vi "Begin.vi"() -> (0 "error out":errorcluster)   [LabVIEW 2013]
doc: "Called before other user functions, this VI is expected to open initial I/O refnums, load in file data, and do all program initialization. Notice that the <B>error out</B> terminal is simply used for data flow. Wiring it to other structures or subVIs ensures that this VI runs first."
uses:
  <vilib>/Rock Robotics/WPI/DriverStation/WPI_DriverStationRobotMode2.ctl
  <vilib>/Rock Robotics/WPI/Joystick/WPI_JoystickDeviceEnum.ctl
  <vilib>/Rock Robotics/SystemInterfaces/DIO/FPGA_DIOPWMChannel.ctl
  <vilib>/Rock Robotics/SystemInterfaces/AI/FPGA_AIGyroChannel.ctl
  <vilib>/Rock Robotics/SystemInterfaces/Typedef/FPGA_TypedefAnalogModuleForGyro.ctl
  <vilib>/Rock Robotics/SystemInterfaces/DIO/FPGA_DIOChannel.ctl
  <vilib>/Rock Robotics/SystemInterfaces/AI/FPGA_AIChannel.ctl
  <vilib>/Rock Robotics/SystemInterfaces/Typedef/FPGA_TypedefAnalogModule.ctl
  <vilib>/Rock Robotics/SystemInterfaces/Typedef/FPGA_TypedefDigitalModule.ctl
  Robot Global Data.vi
  <vilib>/Rock Robotics/WPI/MotorControl/WPI_MotorControlOpen Jaguar.vi
  <vilib>/Rock Robotics/WPI/MotorControl/WPI_MotorControlOpen Victor.vi
  <vilib>/Utility/file.llb/Read From Spreadsheet File (DBL).vi
panel:
  in  "file (use dialog)":path
  out "error out 3":errorcluster
  out "error out 2":errorcluster
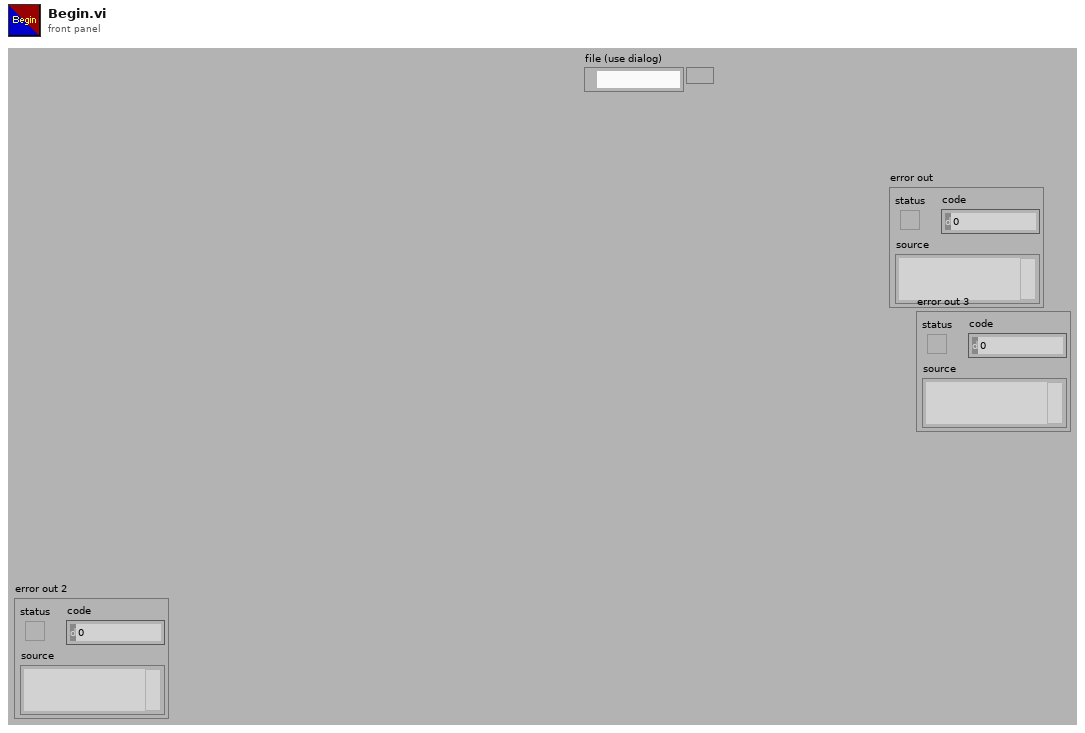
[diagram p1: front panel]
types:
  T1 = typedef "FPGA_TypedefAnalogModule.ctl" = enum16{"Analog Module 1", "Analog Module 2"}
  T2 = typedef "FPGA_AIChannel.ctl" = enum8{"AI 1", "AI 2", "AI 3", "AI 4", "AI 5", "AI 6", "AI 7", "AI 8", "Invalid"}
  T3 = typedef "FPGA_DIOChannel.ctl" = enum8{"DIO 1", "DIO 2", "DIO 3", "DIO 4", "DIO 5", "DIO 6", "DIO 7", "DIO 8", "DIO 9", "DIO 10", "DIO 11", "DIO 12", "DIO 13", "DIO 14", "Invalid"}
  T4 = typedef "FPGA_TypedefDigitalModule.ctl" = enum16{"Digital Module 1", "Digital Module 2"}
  T5 = typedef "FPGA_DIOPWMChannel.ctl" = enum8{"PWM 1", "PWM 2", "PWM 3", "PWM 4", "PWM 5", "PWM 6", "PWM 7", "PWM 8", "PWM 9", "PWM 10", "Invalid"}
  T6 = typedef "WPI_JoystickDeviceEnum.ctl" = enum16{"USB 1", "USB 2", "USB 3", "USB 4", "Kinect 1", "Kinect 2"}
  T7 = typedef "FPGA_TypedefAnalogModuleForGyro.ctl" = enum16{"Analog Module 1"}
  T8 = typedef "FPGA_AIGyroChannel.ctl" = enum8{"AI 1", "AI 2", "Invalid"}
  T9 = typedef "WPI_DriverStationRobotMode2.ctl" = enum16{"Autonomous Disabled", "Autonomous Enabled", "Teleop Disabled", "Teleop Enabled", "Timeout", "Finish", "Test Disabled", "Test Enabled"}
  T10 = typedef "WPI_JoystickDevRef.ctl" = cluster{"Device":T6}
  T11 = typedef "WPI_MotorControlDeviceRef.ctl" = cluster{"DeviceStatus":errorcluster, "Type":enum16{"PWM", "CAN"}, "PWM":cluster{"Digital Module":T4, "PWM Channel":T5, "DeadBand":T12}, "CAN":cluster{"Device Number":u8, "Control Mode":T13, "Semaphore":T14, "Max Vout":dbl}, "Invert":bool, "TransformRef":T15, "InvTransformRef":T15}
  T12 = typedef "WPI_PWMDeadband.ctl" = cluster{"Name":string, "maxPositivePwm":i32, "minPositivePwm":i32, "centerPwm":i32, "maxNegativePwm":i32, "minNegativePwm":i32, "angularRange":u16}
  T13 = typedef "WPI_CANJaguar_ControlMode.ctl" = enum8{"Percent VBus", "Current", "Speed", "Position", "Voltage"}
  T14 = typedef "Semaphore RefNum" = refnum<k1>
  T15 = typedef "WPI_PWMTransform_ConPane.ctl" = refnum<vi>
  T16 = typedef "WPI_ServoDeviceRef.ctl" = cluster{"DeviceStatus":errorcluster, "Digital Module":T4, "PWM Channel":T5, "DeadBand":T12}
  T17 = typedef "WPI_DigitalInputDevRef.ctl" = cluster{"DevStatus":errorcluster, "DIO Channel":T3, "Digital Module":T4}
  T18 = typedef "WPI_AnalogChannelDevRef.ctl" = cluster{"DevStatus":errorcluster, "Analog Module":T1, "Analog Channel":T2}
  T19 = typedef "WPI_GyroDevRef.ctl" = cluster{"DevStatus":errorcluster, "Analog Module":T1, "Analog Channel":T2, "Offset":dbl, "Gain (VoltsPerDegree/Second)":dbl}
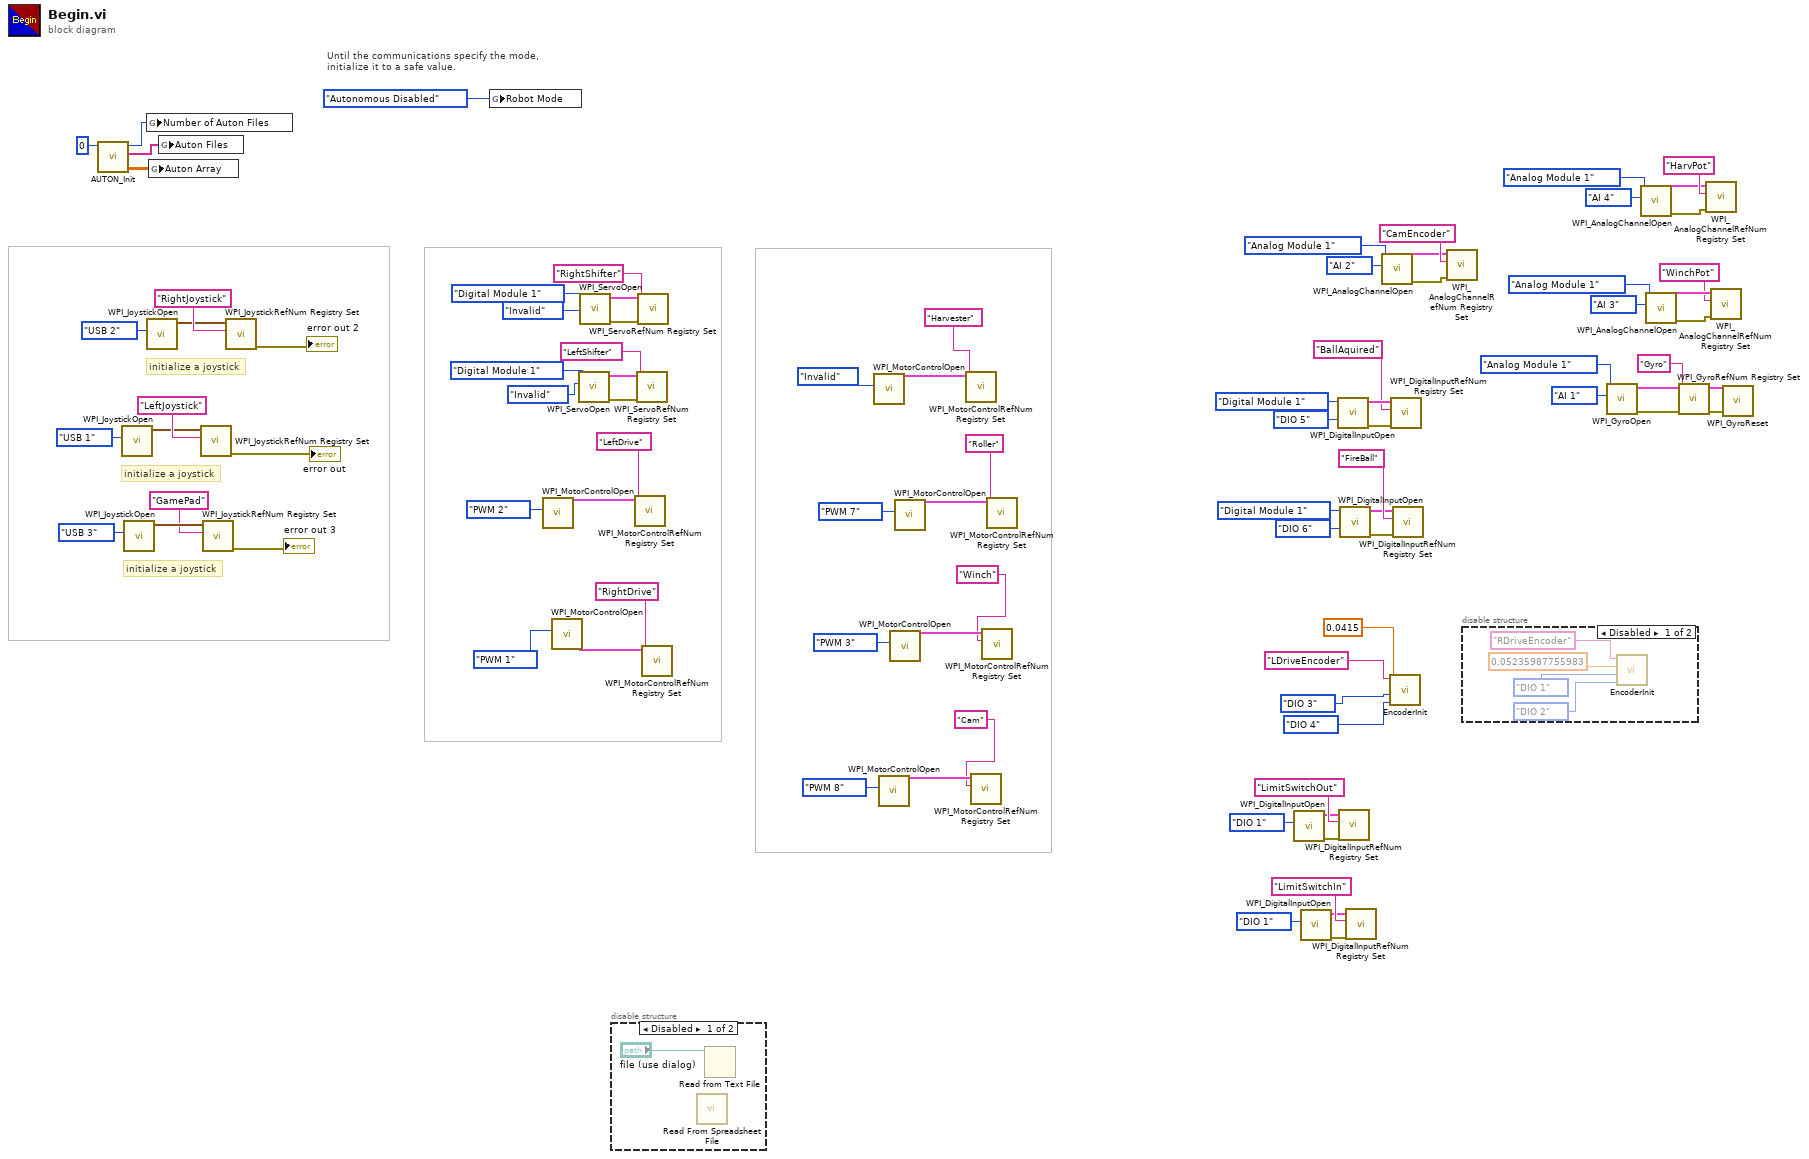
[diagram p0: block diagram]
diagram:
  # "initialize a joystick"
  # "initialize a joystick"
  # "initialize a joystick"
  # "Until the communications specify the mode,\ninitialize it to a safe value."
  n1 = call "AUTON_Init.vi"("Default File"=0) -> ("Auton Array"=w73:dbl[][], "Auton Files"=w72:string[], "Number of Auton Files"=w71:i64)  [unwired: 8 in]
  n2 = call <vilib>:"WPI_JoystickOpen.vi"("JoystickDevice"=WPI_JoystickDeviceEnum."USB 1") -> ("JoystickDevRef"=w87:T10)  [unwired: 10 in]
  n3 = call <vilib>:"WPI_JoystickOpen.vi"("JoystickDevice"=WPI_JoystickDeviceEnum."USB 3") -> ("JoystickDevRef"=w50:T10)  [unwired: 10 in]
  n4 = global write "Robot Global Data.vi" "Number of Auton Files"(w71) -> ()
  n5 = call <vilib>:"WPI_JoystickOpen.vi"("JoystickDevice"=WPI_JoystickDeviceEnum."USB 2") -> ("JoystickDevRef"=w83:T10)  [unwired: 10 in]
  n6 = global write "Robot Global Data.vi" "Auton Array"(w73) -> ()
  n7 = global write "Robot Global Data.vi" "Auton Files"(w72) -> ()
  n8 = call <vilib>:"WPI_JoystickRefNum Registry Set.vi"("refnum name"="LeftJoystick", "JoystickDevRef"=w87) -> ("error out"=→"error out":errorcluster)  [unwired: 8 in, 1 out]
  n9 = call <vilib>:"WPI_JoystickRefNum Registry Set.vi"("refnum name"="GamePad", "JoystickDevRef"=w50) -> ("error out"=→"error out 3":errorcluster)  [unwired: 8 in, 1 out]
  n10 = call <vilib>:"WPI_JoystickRefNum Registry Set.vi"("refnum name"="RightJoystick", "JoystickDevRef"=w83) -> ("error out"=→"error out 2":errorcluster)  [unwired: 8 in, 1 out]
  n11 = global write "Robot Global Data.vi" "Robot Mode"(WPI_DriverStationRobotMode2."Autonomous Disabled" ("Robot Mode")) -> ()
  n12 = call-poly <vilib>:"WPI_MotorControlOpen.vi"("PWM Channel"=FPGA_DIOPWMChannel."PWM 2") -> ("MotorControlDeviceRef"=w79:T11)  [unwired: 9 in, 1 out]
  n13 = call-poly <vilib>:"WPI_MotorControlOpen.vi"("PWM Channel"=FPGA_DIOPWMChannel."PWM 1") -> ("MotorControlDeviceRef"=w76:T11)  [unwired: 9 in, 1 out]
  n14 = call <vilib>:"WPI_ServoOpen.vi"("PWM Channel"=FPGA_DIOPWMChannel."Invalid", "Digital Module (Module 1)"=FPGA_TypedefDigitalModule."Digital Module 1") -> ("error out"=w40:errorcluster, "ServoDeviceRef"=w33:T16)  [unwired: 8 in]
  n15 = call <vilib>:"WPI_ServoOpen.vi"("PWM Channel"=FPGA_DIOPWMChannel."Invalid", "Digital Module (Module 1)"=FPGA_TypedefDigitalModule."Digital Module 1") -> ("error out"=w39:errorcluster, "ServoDeviceRef"=w38:T16)  [unwired: 8 in]
  n16 = disable-structure shown="Disabled" {
    frame Disabled {
      n17 = call-poly <vilib>:"Read From Spreadsheet File.vi"() -> ()  [unwired: 7 in, 5 out]
      n18 = Read from Text File(file (use dialog)="file (use dialog)") -> ()  [unwired: 3 in, 4 out]
    }
    frame Enabled {
    }
  }
  n19 = call <vilib>:"WPI_MotorControlRefNum Registry Set.vi"("refnum name"="LeftDrive", "MotorControlDevRef"=w79) -> ()  [unwired: 8 in, 2 out]
  n20 = call <vilib>:"WPI_ServoRefNum Registry Set.vi"("error in (no error)"=w40, "refnum name"="LeftShifter", "ServoDeviceRef"=w33) -> ()  [unwired: 7 in, 2 out]
  n21 = call <vilib>:"WPI_ServoRefNum Registry Set.vi"("error in (no error)"=w39, "refnum name"="RightShifter", "ServoDeviceRef"=w38) -> ()  [unwired: 7 in, 2 out]
  n22 = call <vilib>:"WPI_MotorControlRefNum Registry Set.vi"("refnum name"="RightDrive", "MotorControlDevRef"=w76) -> ()  [unwired: 8 in, 2 out]
  n23 = call-poly <vilib>:"WPI_MotorControlOpen.vi"("PWM Channel"=FPGA_DIOPWMChannel."Invalid") -> ("MotorControlDeviceRef"=w69:T11)  [unwired: 9 in, 1 out]
  n24 = call-poly <vilib>:"WPI_MotorControlOpen.vi"("PWM Channel"=FPGA_DIOPWMChannel."PWM 8") -> ("MotorControlDeviceRef"=w18:T11)  [unwired: 9 in, 1 out]
  n25 = call-poly <vilib>:"WPI_MotorControlOpen.vi"("PWM Channel"=FPGA_DIOPWMChannel."PWM 3") -> ("MotorControlDeviceRef"=w20:T11)  [unwired: 9 in, 1 out]
  n26 = call-poly <vilib>:"WPI_MotorControlOpen.vi"("PWM Channel"=FPGA_DIOPWMChannel."PWM 7") -> ("MotorControlDeviceRef"=w66:T11)  [unwired: 9 in, 1 out]
  n27 = call <vilib>:"WPI_MotorControlRefNum Registry Set.vi"("refnum name"="Harvester", "MotorControlDevRef"=w69) -> ()  [unwired: 8 in, 2 out]
  n28 = call <vilib>:"WPI_MotorControlRefNum Registry Set.vi"("refnum name"="Cam", "MotorControlDevRef"=w18) -> ()  [unwired: 8 in, 2 out]
  n29 = call <vilib>:"WPI_MotorControlRefNum Registry Set.vi"("refnum name"="Winch", "MotorControlDevRef"=w20) -> ()  [unwired: 8 in, 2 out]
  n30 = call <vilib>:"WPI_MotorControlRefNum Registry Set.vi"("refnum name"="Roller", "MotorControlDevRef"=w66) -> ()  [unwired: 8 in, 2 out]
  n31 = call <vilib>:"WPI_DigitalInputOpen.vi"("DIO Channel"=FPGA_DIOChannel."DIO 1") -> ("error out"=w22:errorcluster, "DigitalInputDevRef"=w23:T17)  [unwired: 9 in]
  n32 = call <vilib>:"WPI_DigitalInputOpen.vi"("DIO Channel"=FPGA_DIOChannel."DIO 1") -> ("error out"=w25:errorcluster, "DigitalInputDevRef"=w26:T17)  [unwired: 9 in]
  n33 = call <vilib>:"WPI_DigitalInputOpen.vi"("DIO Channel"=FPGA_DIOChannel."DIO 5", "Digital Module (Module 1)"=FPGA_TypedefDigitalModule."Digital Module 1") -> ("error out"=w60:errorcluster, "DigitalInputDevRef"=w59:T17)  [unwired: 8 in]
  n34 = call <vilib>:"WPI_DigitalInputRefNum Registry Set.vi"("error in (no error)"=w22, "refnum name"="LimitSwitchOut", "DigitalInputDevRef"=w23) -> ()  [unwired: 7 in, 2 out]
  n35 = call <vilib>:"WPI_DigitalInputOpen.vi"("DIO Channel"=FPGA_DIOChannel."DIO 6", "Digital Module (Module 1)"=FPGA_TypedefDigitalModule."Digital Module 1") -> ("error out"=w6:errorcluster, "DigitalInputDevRef"=w7:T17)  [unwired: 8 in]
  n36 = call <vilib>:"WPI_DigitalInputRefNum Registry Set.vi"("error in (no error)"=w25, "refnum name"="LimitSwitchIn", "DigitalInputDevRef"=w26) -> ()  [unwired: 7 in, 2 out]
  n37 = call <vilib>:"WPI_AnalogChannelOpen.vi"("Analog Channel"=FPGA_AIChannel."AI 2", "Analog Module (Module 1)"=FPGA_TypedefAnalogModule."Analog Module 1") -> ("error out"=w12:errorcluster, "AIDeviceRef"=w11:T18)  [unwired: 8 in]
  n38 = call "EncoderInit.vi"("refnum name"="LDriveEncoder", "DistancePerCount"=0.0415, "DIO Channel"=FPGA_DIOChannel."DIO 3", "DIO Channel 2"=FPGA_DIOChannel."DIO 4") -> ()  [unwired: 7 in]
  n39 = call <vilib>:"WPI_DigitalInputRefNum Registry Set.vi"("error in (no error)"=w60, "refnum name"="BallAquired", "DigitalInputDevRef"=w59) -> ()  [unwired: 7 in, 2 out]
  n40 = call <vilib>:"WPI_DigitalInputRefNum Registry Set.vi"("error in (no error)"=w6, "refnum name"="FireBall", "DigitalInputDevRef"=w7) -> ()  [unwired: 7 in, 2 out]
  n41 = call <vilib>:"WPI_AnalogChannelRefNum Registry Set.vi"("error in (no error)"=w12, "refnum name"="CamEncoder", "AIDeviceRef"=w11) -> ()  [unwired: 7 in, 2 out]
  n42 = disable-structure shown="Disabled" {
    frame Disabled {
      n43 = call "EncoderInit.vi"("refnum name"="RDriveEncoder", "DistancePerCount"=0.05235987755983, "DIO Channel"=FPGA_DIOChannel."DIO 1", "DIO Channel 2"=FPGA_DIOChannel."DIO 2") -> ()  [unwired: 7 in]
    }
    frame Enabled {
    }
  }
  n44 = call <vilib>:"WPI_GyroOpen.vi"("Analog Channel"=FPGA_AIGyroChannel."AI 1", "Analog Module (Module 1)"=FPGA_TypedefAnalogModuleForGyro."Analog Module 1") -> ("error out"=w53:errorcluster, "GyroDevRef"=w63:T19)  [unwired: 7 in, 1 out]
  n45 = call <vilib>:"WPI_AnalogChannelOpen.vi"("Analog Channel"=FPGA_AIChannel."AI 4", "Analog Module (Module 1)"=FPGA_TypedefAnalogModule."Analog Module 1") -> ("error out"=w2:errorcluster, "AIDeviceRef"=w1:T18)  [unwired: 8 in]
  n46 = call <vilib>:"WPI_AnalogChannelOpen.vi"("Analog Channel"=FPGA_AIChannel."AI 3", "Analog Module (Module 1)"=FPGA_TypedefAnalogModule."Analog Module 1") -> ("error out"=w47:errorcluster, "AIDeviceRef"=w48:T18)  [unwired: 8 in]
  n47 = call <vilib>:"WPI_GyroRefNum Registry Set.vi"("error in (no error)"=w53, "refnum name"="Gyro", "GyroDevRef"=w63) -> ("error out"=w54:errorcluster, "GyroDevRef"=w55:T19)  [unwired: 7 in]
  n48 = call <vilib>:"WPI_AnalogChannelRefNum Registry Set.vi"("error in (no error)"=w2, "refnum name"="HarvPot", "AIDeviceRef"=w1) -> ()  [unwired: 7 in, 2 out]
  n49 = call <vilib>:"WPI_AnalogChannelRefNum Registry Set.vi"("error in (no error)"=w47, "refnum name"="WinchPot", "AIDeviceRef"=w48) -> ()  [unwired: 7 in, 2 out]
  n50 = call <vilib>:"WPI_GyroReset.vi"("error in (no error)"=w54, "GyroDevRef"=w55) -> ()  [unwired: 8 in, 2 out]
